vi "PythonScriptsTest.vi"() -> ()   [LabVIEW 2020]
panel:
  in  "working directory":path=path "/home/pi"
  in  "command line":string="python save.py test.png "
  out "standard error":string
  out "return code":i32
  out "standard output":string
  # "Команды для отладки и переноса файлов\nfdisk -l  - проверка активных устройств\nmount /dev/sda1 /media/usb - Монтирование флешки /dev/sda1 в директорию /media/usb\numount /dev/sda1 /media/usb - Размонтирование флешки /dev/sda1 из директории /media/usb\npython save.py test.png - запуск скрипта для сохранения изображения с камеры с названием файла test.png\ncat result.txt - считывание result.txt файла\npython camera.py 1.png 2.png 3.png 4.png - анализ доски заказов"
  # "1px -0,714mm"
  # "python cv.py F 7__.png 50"
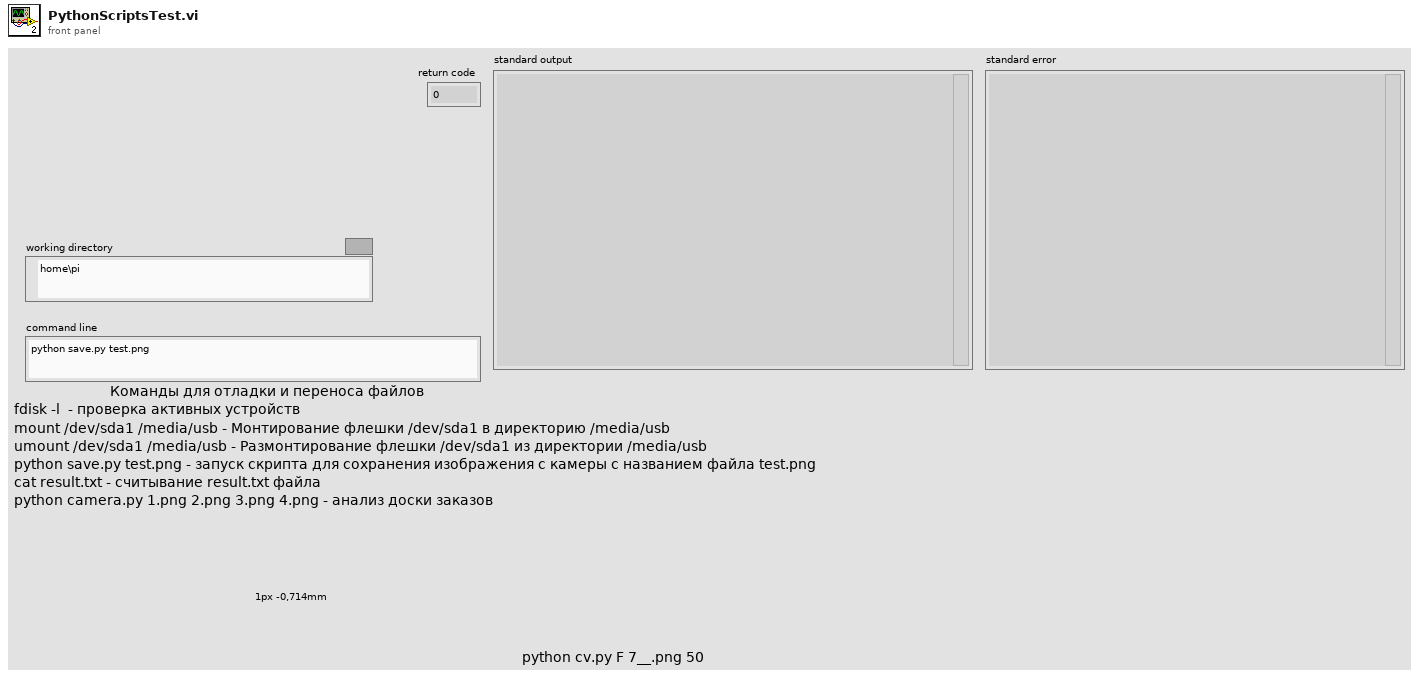
[diagram p1: front panel]
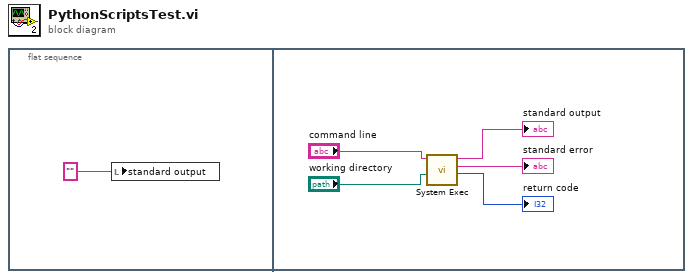
[diagram p0: block diagram]
diagram:
  n1 = flat-sequence {
    frame #0 {
      n2 = local write "standard output"("" ("standard output")) -> ()
    }
    frame #1 {
      n3 = call <vilib>:"System Exec.vi"("working directory"="working directory", "command line"="command line") -> ("return code"=→"return code":i32, "standard error"=→"standard error":string, "standard output"=→"standard output":string)  [unwired: 6 in, 1 out]
    }
  }
